vi "Set On Off.vi"(8 "error in (no error)":errorcluster, 10 "on-off":bool, 11 "simple Class in":refnum<class "Simple Class.lvclass">) -> (0 "error out":errorcluster, 3 "simple Class out":refnum<class "Simple Class.lvclass">)   [LabVIEW 2023, in "Simple Class.lvclass"]
doc: "Set \"on-off.\""
uses:
  Simple Class.lvclass
  Simple Class.lvclass/Simple Class.ctl
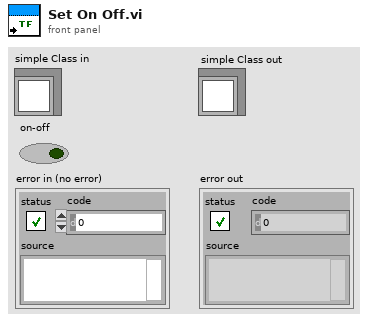
[diagram p1: front panel]
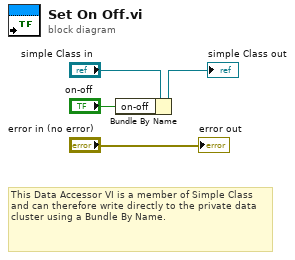
[diagram p0: block diagram]
diagram:
  # "This Data Accessor VI is a member of Simple Class and can therefore write directly to the private data cluster using a Bundle By Name."
  n1 = Bundle By Name(cluster="simple Class in", "on-off"="on-off") -> (→"simple Class out":refnum<class "Simple Class.lvclass">)
  "error out" <- "error in (no error)"
